vi "Read Scan Direction.vi"(8 "error in (no error)":errorcluster, 11 "Galvonometer in":refnum<class "Galvonometer.lvclass">) -> (0 "error out":errorcluster, 2 "Scan Direction":string(combo)="Azimuth (X)", 3 "Galvonometer out":refnum<class "Galvonometer.lvclass">)   [LabVIEW 2017, in "Galvonometer.lvclass"]
uses:
  Galvonometer.lvclass
  Galvonometer.lvclass/Galvonometer.ctl
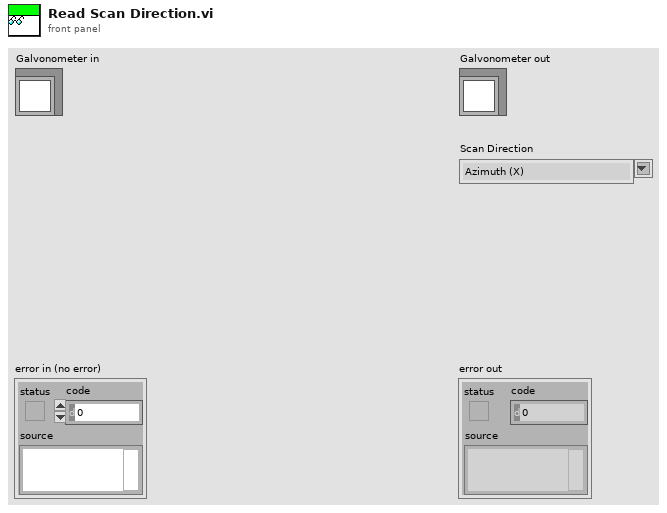
[diagram p1: front panel]
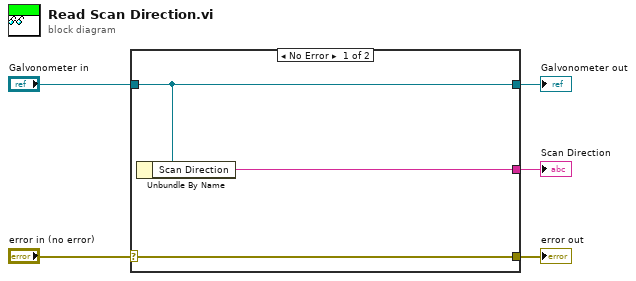
[diagram p0: block diagram]
diagram:
  n1 = case shown="No Error" "error in (no error)" {
    selector: "error in (no error)" -> [w8 w9]
    tunnel: [w8 w9] -> w4
    tunnel: [w7 w10] -> w2
    tunnel: "Galvonometer in" -> [w7 w10]
    tunnel: [w6 _] -> w1
    frame No Error {
      n2 = Unbundle By Name(w7) -> ("Scan Direction"=w6:string)
    }
    frame Error {
    }
  }
  "error out" <- w4
  "Galvonometer out" <- w2
  "Scan Direction" <- w1
